vi "test.vi"() -> ()   [LabVIEW 2010, in "GenericStage.lvclass"]
uses:
  GenericStage.lvclass
  main/labview_source/type_definitions/clusters/controls_refs.ctl
  common/classes/SpaceVector/SpaceVector/SpaceVector.lvclass
  translation_mode_enum.ctl
  common/classes/GenericComponent/GenericComponent/GenericComponent.lvclass
  common/clusters/plugin_specification.ctl
panel:
  in  "configuration":string(combo)
  in  "create button":bool
  in  "move relative":bool
  in  "move":bool
  in  "y":dbl[unit]
  in  "z":dbl[unit]
  in  "x":dbl[unit]
  in  "component path":path
  in  "stop":bool
  # "Stage test"
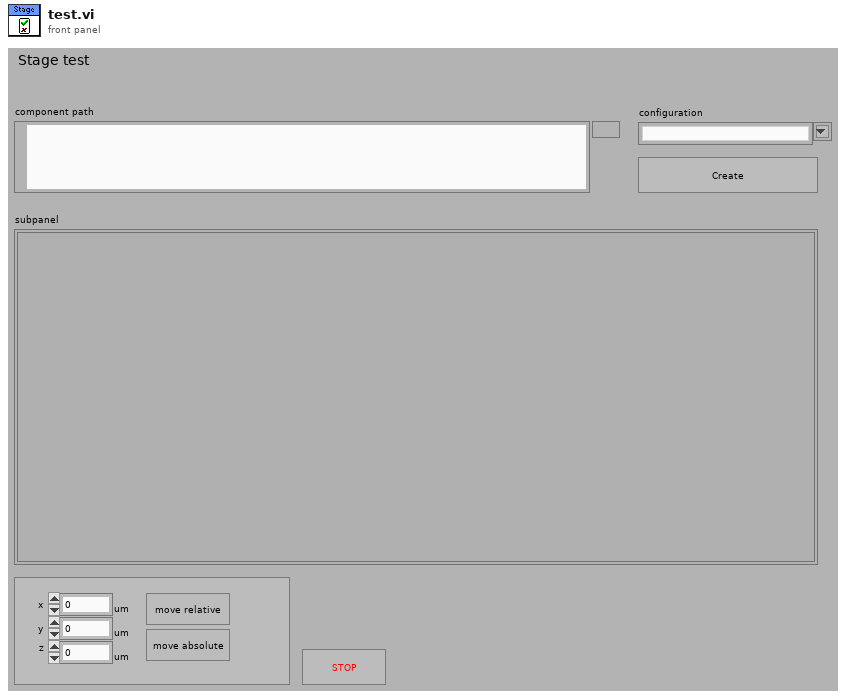
[diagram p1: front panel]
types:
  T1 = typedef "plugin_specification.ctl" = cluster{"class path":string, "configuration":string, "label":string, "settings name":string}
  T2 = typedef "controls_refs.ctl" = cluster{"scan start button":refnum<vi>, "tabs":cluster{"main":refnum<vi>, "settings":refnum<vi>}, "subpanels":cluster{"imagingMode":refnum<vi>, "scanHead":refnum<vi>, "display":refnum<vi>, "experimentController":refnum<vi>, "instrument":refnum<vi>, "stage":refnum<vi>, "stimulator":refnum<vi>, "dataCollection":refnum<vi>, "analyser":refnum<vi>, "daq":refnum<vi>, "imageAssembler":refnum<vi>}, "drop-downs":cluster{"run mode":refnum<vi>, "imagingMode":refnum<vi>, "experimentalController":refnum<vi>, "objective":refnum<vi>}, "status lights":cluster{"experimentController":refnum<vi>, "imagingMode":refnum<vi>, "scanHead":refnum<vi>, "daq":refnum<vi>, "imageAssembler":refnum<vi>, "dataCollection":refnum<vi>, "display":refnum<vi>, "analyser":refnum<vi>, "stage":refnum<vi>, "stimulator":refnum<vi>, "instrument":refnum<vi>}, "message":refnum<vi>, "stimulator enabled?":refnum<vi>, "saving":cluster{"data folder path":refnum<vi>, "file base name":refnum<vi>, "notebook":refnum<vi>}, "progress bar":refnum<vi>, "update icon":refnum<vi>, "title":refnum<vi>, "main vi":refnum<vi>, "user":refnum<vi>, "exit_button":refnum<vi>, "CPU usage %":refnum<vi>}
  T3 = typedef "GenericStage.lvclass/translation_mode_enum.ctl" = enum16{"DON'T MOVE", "relative", "absolute"}
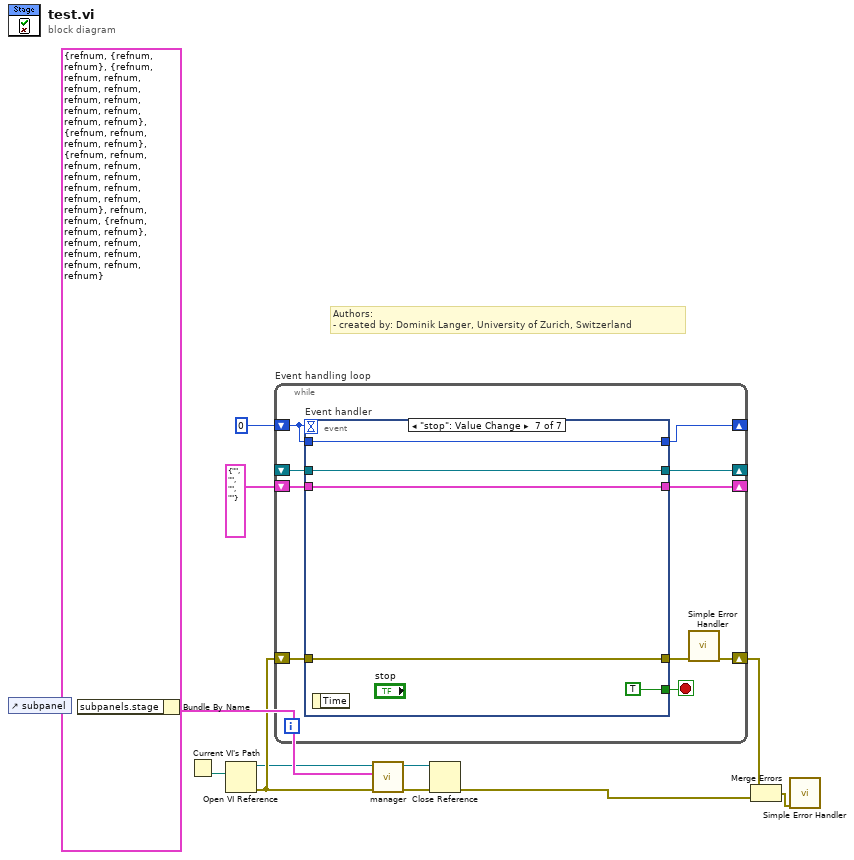
[diagram p0: block diagram]
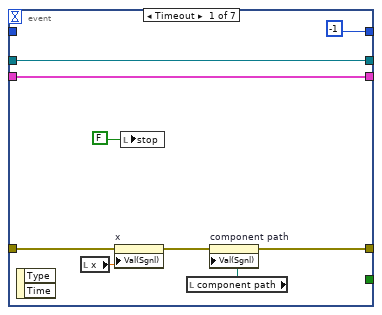
[diagram p2: hidden frame]
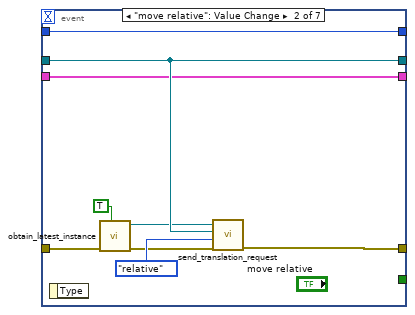
[diagram p3: hidden frame]
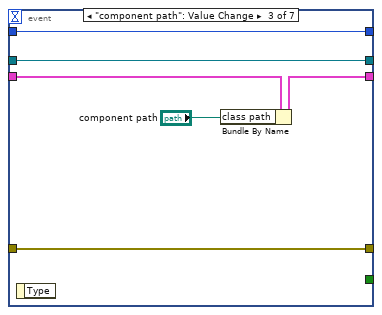
[diagram p4: hidden frame]
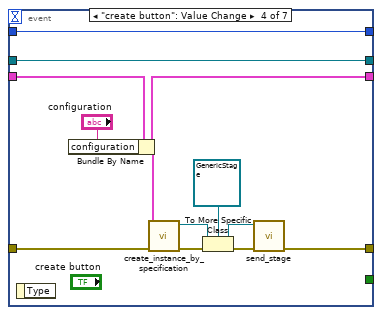
[diagram p5: hidden frame]
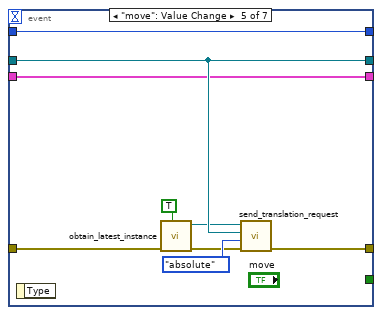
[diagram p6: hidden frame]
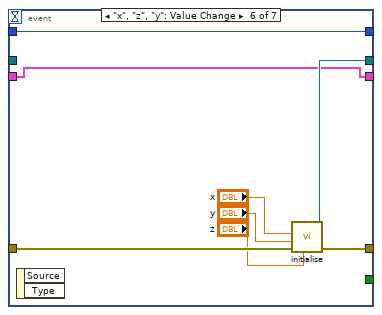
[diagram p7: hidden frame]
diagram:
  # "Authors: \n- created by: Dominik Langer, University of Zurich, Switzerland"
  n1 = control-ref of="subpanel"() -> (w12:refnum<vi>)
  n2 = Bundle By Name(cluster=T2 {"scan start button"=refnum, "tabs"={"main"=refnum, "settings"=refnum}, "subpanels"={"imagingMode"=refnum, "scanHead"=refnum, "display"=refnum, "experimentController"=refnum, "instrument"=refnum, "stage"=refnum, "stimulator"=refnum, "dataCollection"=refnum, "analyser"=refnum, "daq"=refnum, "imageAssembler"=refnum}, "drop-downs"={"run mode"=refnum, "imagingMode"=refnum, "experimentalController"=refnum, "objective"=refnum}, "status lights"={"experimentController"=refnum, "imagingMode"=refnum, "scanHead"=refnum, "daq"=refnum, "imageAssembler"=refnum, "dataCollection"=refnum, "display"=refnum, "analyser"=refnum, "stage"=refnum, "stimulator"=refnum, "instrument"=refnum}, "message"=refnum, "stimulator enabled?"=refnum, "saving"={"data folder path"=refnum, "file base name"=refnum, "notebook"=refnum}, "progress bar"=refnum, "update icon"=refnum, "title"=refnum, "main vi"=refnum, "user"=refnum, "exit_button"=refnum, "CPU usage %"=refnum} ("control references"), "subpanels.stage"=w12) -> (w11:T2)
  n3 = Current VI's Path() -> (path=w7:path)
  n4 = Open VI Reference(vi path=w7) -> (vi reference=w5:refnum<vi>, error out=w6:errorcluster)  [unwired: 5 in]
  n5 = while "Event handling loop" {
    shift-right: [w14] -> w9
    shift-left: w6 -> [w23]
    shift-right: [w21] -> _
    shift-left: 0 -> [w22]
    shift-right: [w20] -> _
    shift-left: _ -> [w19]
    shift-right: [w18] -> _
    shift-left: T1 {"class path"="", "configuration"="", "label"="", "settings name"=""} ("component specification") -> [w17]
    stop <- w16 stop-if-true
    n6 = event "Event handler" shown="[6] \"stop\": Value Change" {
      selector: _ -> [_ _ _ _ _ _ _]
      dyn-events: _ -> [_ _ _ _ _ _ _]
      timeout: w22 -> [_ _ _ _ _ _ _]
      tunnel: [_ _ _ _ _ _ TRUE] -> w16
      tunnel: w23 -> [w25 w36 w46 w57 w63 w75 w79]
      tunnel: w22 -> [_ w41 w47 w59 w68 w76 w80]
      tunnel: [-1 w41 w47 w59 w68 w76 w80] -> w21
      tunnel: [w28 w40 w46 w49 w67 w74 w79] -> w15
      tunnel: [w30 w38 w45 w58 w66 w70 w78] -> w20
      tunnel: w19 -> [w30 w38 w45 w58 w66 _ w78]
      tunnel: [w29 w37 w42 w54 w64 w69 w77] -> w18
      tunnel: w17 -> [w29 w37 w44 w55 w64 w69 w77]
      event Timeout {
        n7 = event-data() -> ()  [unwired: 3 out]
        n8 = local read "x"() -> (w26:dbl[unit])
        n9 = property on="x" class="DigNum (strict)"(error in=w25, "Val(Sgnl)"=w26) -> (error out=w24:errorcluster)  [unwired: 1 in, 1 out]
        n10 = local write "stop"(FALSE) -> ()
        n11 = local read "component path"() -> (w27:path)
        n12 = property on="component path" class="Path"(error in=w24, "Val(Sgnl)"=w27) -> (error out=w28:errorcluster)  [unwired: 1 in, 1 out]
      }
      event "move relative": Value Change {
        n13 = event-data() -> ()  [unwired: 2 out]
        n14 = call "obtain_latest_instance.vi"("quick, but maybe outdated?"=TRUE, "error in (no error)"=w36) -> ("error out"=w35:errorcluster, "GenericStage out"=w34:refnum<class "GenericStage.lvclass">)  [unwired: 8 in]
        n15 = call-dynamic "send_translation_request.vi"("error in (no error)"=w35, "translation mode"=translation_mode_enum."relative", "translation vector"=w38, "GenericStage in"=w34) -> ("error out"=w40:errorcluster)  [unwired: 7 out]
      }
      event "component path": Value Change {
        n16 = event-data() -> ()  [unwired: 2 out]
        n17 = Bundle By Name(cluster=w44, "class path"="component path") -> (w42:T1)
      }
      event "create button": Value Change {
        n18 = event-data() -> ()  [unwired: 2 out]
        n19 = Bundle By Name(cluster=w55, "configuration"="configuration") -> (w54:T1)
        n20 = call "create_instance_by_specification.vi"("error in (no error)"=w57, "component specification"=w54) -> ("error out"=w52:errorcluster, "GenericPlugin out"=w51:refnum<class "GenericComponent.lvclass">)  [unwired: 7 in, 1 out]
        n21 = To More Specific Class(target class=refnum<class "GenericStage.lvclass"> refnum ("GenericStage.lvclass"), reference=w51, error in=w52) -> (specific class reference=w48:refnum<class "GenericStage.lvclass">, error out=w50:errorcluster)
        n22 = call-dynamic "send_stage.vi"("error in (no error)"=w50, "GenericStage in"=w48) -> ("error out"=w49:errorcluster)  [unwired: 8 in, 1 out]
      }
      event "move": Value Change {
        n23 = event-data() -> ()  [unwired: 2 out]
        n24 = call "obtain_latest_instance.vi"("quick, but maybe outdated?"=TRUE, "error in (no error)"=w63) -> ("error out"=w62:errorcluster, "GenericStage out"=w60:refnum<class "GenericStage.lvclass">)  [unwired: 8 in]
        n25 = call-dynamic "send_translation_request.vi"("error in (no error)"=w62, "translation mode"=translation_mode_enum."absolute", "translation vector"=w66, "GenericStage in"=w60) -> ("error out"=w67:errorcluster)  [unwired: 7 out]
      }
      event "x", "z", "y": Value Change {
        n26 = event-data() -> ()  [unwired: 3 out]
        n27 = call "initialise.vi"("z"="z", "error in (no error)"=w75, "y"="y", "x"="x") -> ("error out"=w74:errorcluster, "SpaceVector out"=w70:refnum<class "SpaceVector.lvclass">)  [unwired: 6 out]
      }
      event "stop": Value Change {
        n28 = event-data() -> ()  [unwired: 2 out]
      }
    }
    n29 = call <vilib>:"Simple Error Handler.vi"("error in (no error)"=w15) -> ("error out"=w14:errorcluster)  [unwired: 4 in, 4 out]
  }
  n30 = call "manager.vi"("error in (no error)"=w6, "control references"=w11, "top-level VI ref in"=w5) -> ("error out"=w4:errorcluster, "top-level VI ref out"=w2:refnum<vi>)  [unwired: 7 in]
  n31 = Close Reference(reference=w2, error in (no error)=w4) -> (error out=w3:errorcluster)
  n32 = Merge Errors(w9, w3) -> (w1:errorcluster)
  n33 = call <vilib>:"Simple Error Handler.vi"("error in (no error)"=w1) -> ()  [unwired: 4 in, 5 out]
